vi "Append Path.vi"(10 "Item Name":string, 11 "Parent Path":string) -> (3 "Path":string)   [LabVIEW 2020, in "Negentropic IDE.lvlib"]
uses:
  Negentropic IDE.lvlib
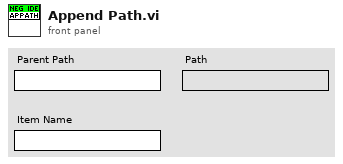
[diagram p1: front panel]
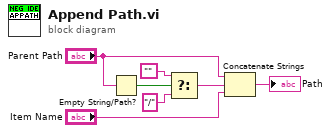
[diagram p0: block diagram]
diagram:
  n1 = Empty String/Path?(string/path="Parent Path") -> (empty?=w7:bool)
  n2 = Select(t="", s=w7, f="/") -> (s? t:f=w4:string)
  n3 = Concatenate Strings("Parent Path", w4, "Item Name") -> (→"Path":string)
